vi "ROS_Status_Publisher.vi"() -> ()   [LabVIEW 2016]
uses:
  <userlib>/ROS for LabVIEW Software/ROS/Code/Console/Servers/ServerSubs/TopicDef.ctl
  <userlib>/ROS for LabVIEW Software/ROS/Code/SubVIs/_ROSDirection.ctl
  GlobalVI.vi
  <userlib>/ROS for LabVIEW Software/ROS/MessageBuilding/std_msgs/subs/stringScalar.vi
  <userlib>/ROS for LabVIEW Software/ROS/Code/_ROSDefinition.vi
panel:
  out "ROS Write ERR":errorcluster
  out "JSON string 2":string
  out "error out":errorcluster
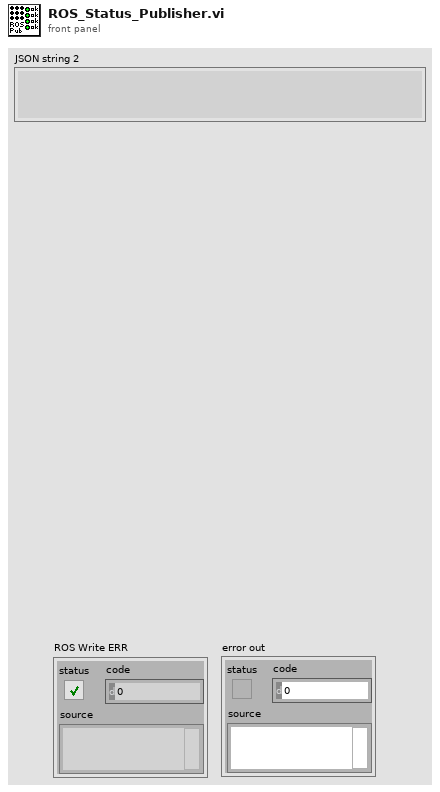
[diagram p1: front panel]
types:
  T1 = typedef "TopicDef.ctl" = cluster{"Topic":string, "Type":string, "Action":T2, "Update (ms)":u16, "queue size":u16}
  T2 = typedef "_ROSDirection.ctl" = enum16{"Node", "Publisher", "Subscriber", "ServiceClient", "ServiceProvider"}
  T3 = typedef "_ROSControl.ctl" = cluster{"topic port":u16, "Node":string, "topic":string, "type":string, "node port":u16, "error ":errorcluster, "Direction":T2, "Update (ms)":u16, "FIFO size":u16}
  T4 = cluster{"status":cluster{"liftStatus":bool, "lidarBackStatus":bool, "uwbStatus":bool, "lightStatus":bool, "liftState":i32, "uwbPosition":cluster{"x":dbl, "y":dbl, "z":dbl}, "distance":sgl}}
  T5 = cluster{"liftStatus":bool, "lidarBackStatus":bool, "uwbStatus":bool, "lightStatus":bool, "currentLiftState":i32, "position":cluster{"x":dbl, "y":dbl, "z":dbl}, "avgDist":sgl}
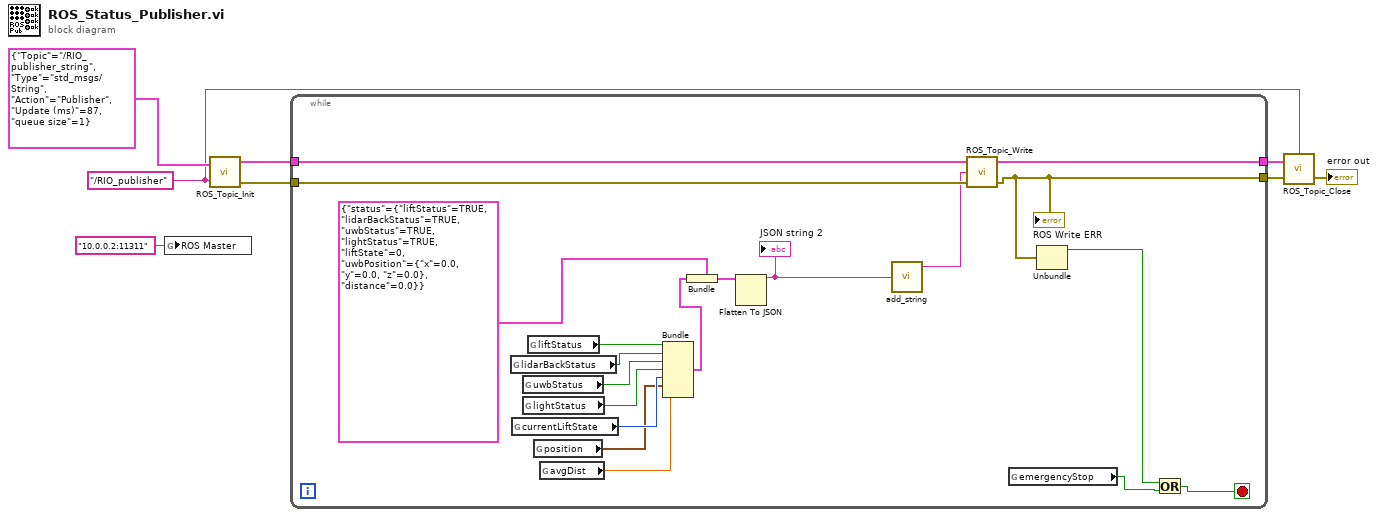
[diagram p0: block diagram]
diagram:
  w7 = "/RIO_publisher" ("node")
  n1 = global write "_ROSDefinition.vi" "ROS Master"("10.0.0.2:11311" ("ROS Master")) -> ()
  n2 = call <userlib>:"ROS_Topic_Init.vi"("Definitions"=T1 {"Topic"="/RIO_publisher_string", "Type"="std_msgs/String", "Action"=enum."Publisher", "Update (ms)"=87, "queue size"=1}, "node"=w7) -> ("ROS out"=w6:T3, "error out"=w4:errorcluster)  [unwired: 1 in]
  n3 = while {
    tunnel: w6 -> [w27]
    tunnel: [w26] -> w5
    tunnel: w4 -> [w25]
    tunnel: [w12] -> w3
    stop <- w9 stop-if-true
    n4 = global read "GlobalVI.vi" "lidarBackStatus"() -> (w22:bool)
    n5 = global read "GlobalVI.vi" "currentLiftState"() -> (w20:i32)
    n6 = global read "GlobalVI.vi" "uwbStatus"() -> (w23:bool)
    n7 = global read "GlobalVI.vi" "lightStatus"() -> (w24:bool)
    n8 = global read "GlobalVI.vi" "liftStatus"() -> (w21:bool)
    n9 = global read "GlobalVI.vi" "position"() -> (w19:cluster{"x":dbl, "y":dbl, "z":dbl})
    n10 = global read "GlobalVI.vi" "avgDist"() -> (w18:sgl)
    n11 = Bundle("liftStatus"=w21, "lidarBackStatus"=w22, "uwbStatus"=w23, "lightStatus"=w24, "currentLiftState"=w20, "position"=w19, "avgDist"=w18) -> (w16:T5)  [unwired: 1 in]
    n12 = Bundle(cluster=T4 {"status"={"liftStatus"=TRUE, "lidarBackStatus"=TRUE, "uwbStatus"=TRUE, "lightStatus"=TRUE, "liftState"=0, "uwbPosition"={"x"=0.0, "y"=0.0, "z"=0.0}, "distance"=0.0}}, "status"=w16) -> (w15:T4)
    n13 = Flatten To JSON(anything=w15) -> (JSON string=w13:string)  [unwired: 2 in, 1 out]
    "JSON string 2" <- w13
    n14 = call-poly <userlib>:"add_string.vi"("String"=w13) -> ("msg out"=w14:string)  [unwired: 4 in]
    n15 = call <userlib>:"ROS_Topic_Write.vi"("error in (no error)"=w25, "Msg in"=w14, "ROS in"=w27) -> ("error out"=w12:errorcluster, "ROS out"=w26:T3)  [unwired: 1 in]
    "ROS Write ERR" <- w12
    n16 = global read "GlobalVI.vi" "emergencyStop"() -> (w11:bool)
    n17 = Unbundle(w12) -> ("status"=w10:bool)  [unwired: 2 out]
    n18 = Or(x=w10, y=w11) -> (x .or. y?=w9:bool)
  }
  n19 = call <userlib>:"ROS_Topic_Close.vi"("error in"=w3, "ROS in"=w5, "node"=w7) -> ("error out"=→"error out":errorcluster)  [unwired: 1 in]
